vi "example_getSelectedWires.vi"() -> ()   [LabVIEW 2023]
uses:
  TLC_Scripto.lvlib
  BlockDiagram/BlockDiagram.lvclass
  Wire/Wire.lvclass
panel:
  in  "mode":enum16{"TopMostBlockDiagram", "LoadVI"}(ring)
  out "wires":refnum<class "Wire.lvclass">[](array[class])
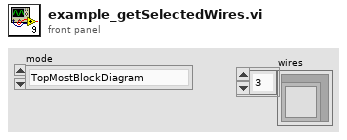
[diagram p1: front panel]
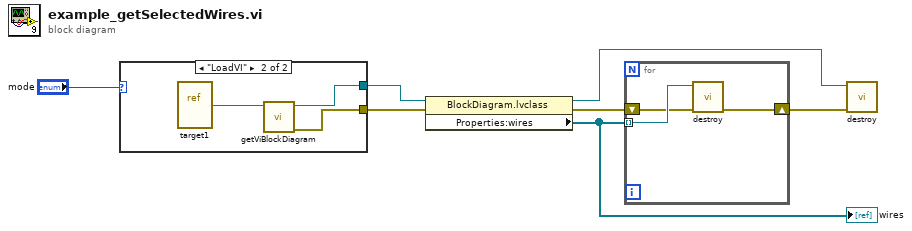
[diagram p0: block diagram]
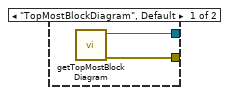
[diagram p2: hidden frame]
diagram:
  n1 = case shown="\"LoadVI\"" "mode" {
    tunnel: [w9 w12] -> w7
    tunnel: [w8 w11] -> w5
    frame "TopMostBlockDiagram", Default {
      n2 = call "getTopMostBlockDiagram.vi"() -> ("error out"=w8:errorcluster, "topMostBlockDiagram"=w9:refnum<class "BlockDiagram.lvclass">)  [unwired: 10 in]
    }
    frame "LoadVI" {
      n3 = vi-ref "target1.vi"() -> (w10:refnum<vi>)
      n4 = call "getViBlockDiagram.vi"("ViRef"=w10) -> ("error out"=w11:errorcluster, "topMostBlockDiagram"=w12:refnum<class "BlockDiagram.lvclass">)  [unwired: 9 in]
    }
  }
  n5 = property class="BlockDiagram.lvclass"(reference=w7, error in=w5) -> (reference out=w4:refnum<class "BlockDiagram.lvclass">, error out=w2:errorcluster, "Properties:wires"=w3:refnum<class "Wire.lvclass">[])
  "wires" <- w3
  n6 = for {
    tunnel: w3 -> [w15] mode=indexing
    shift-right: [w13] -> w1
    shift-left: w2 -> [w14]
    n7 = call-dynamic "destroy.vi"("Error In"=w14, "Generic In"=w15) -> ("Error Out"=w13:errorcluster)  [unwired: 9 in]
  }
  n8 = call-dynamic "destroy.vi"("Error In"=w1, "Generic In"=w4) -> ()  [unwired: 9 in, 1 out]
